vi "Main.vi"() -> ()   [LabVIEW 2020]
panel:
  out "Processed Stream":T1(plugin-control)
  out "Cat 6":dbl(slide) caption="40cm<" scale=0.0..100.0 scale format="%#.3f"
  out "Cat 5":dbl(slide) caption="30-40cm" scale=0.0..100.0 scale format="%#.3f"
  out "Cat 4":dbl(slide) caption="15-30cm" scale=0.0..100.0 scale format="%#.3f"
  out "Cat 3":dbl(slide) caption="10-15cm" scale=0.0..100.0 scale format="%#.3f"
  out "Cat 2":dbl(slide) caption="5-10cm" scale=0.0..100.0 scale format="%#.3f"
  out "Cat 1":dbl(slide) caption="0-5cm" scale=0.0..100.0 scale format="%#.3f"
  out "Live Stream":T1(plugin-control)
  out "Date & Time":string
  in  "Abort":bool
  in  "Maintenance":bool
  in  "Setting":bool
  in  "Report":bool
  in  "Parameters":bool
  in  "Login":bool
  out "Errors":bool
  out "Warnings":bool
  out "Reject Alarm":bool
  out "Sampler Signal":bool
  out "System Unready":bool
  out "System Ready":bool
  # "Smart Grading System"
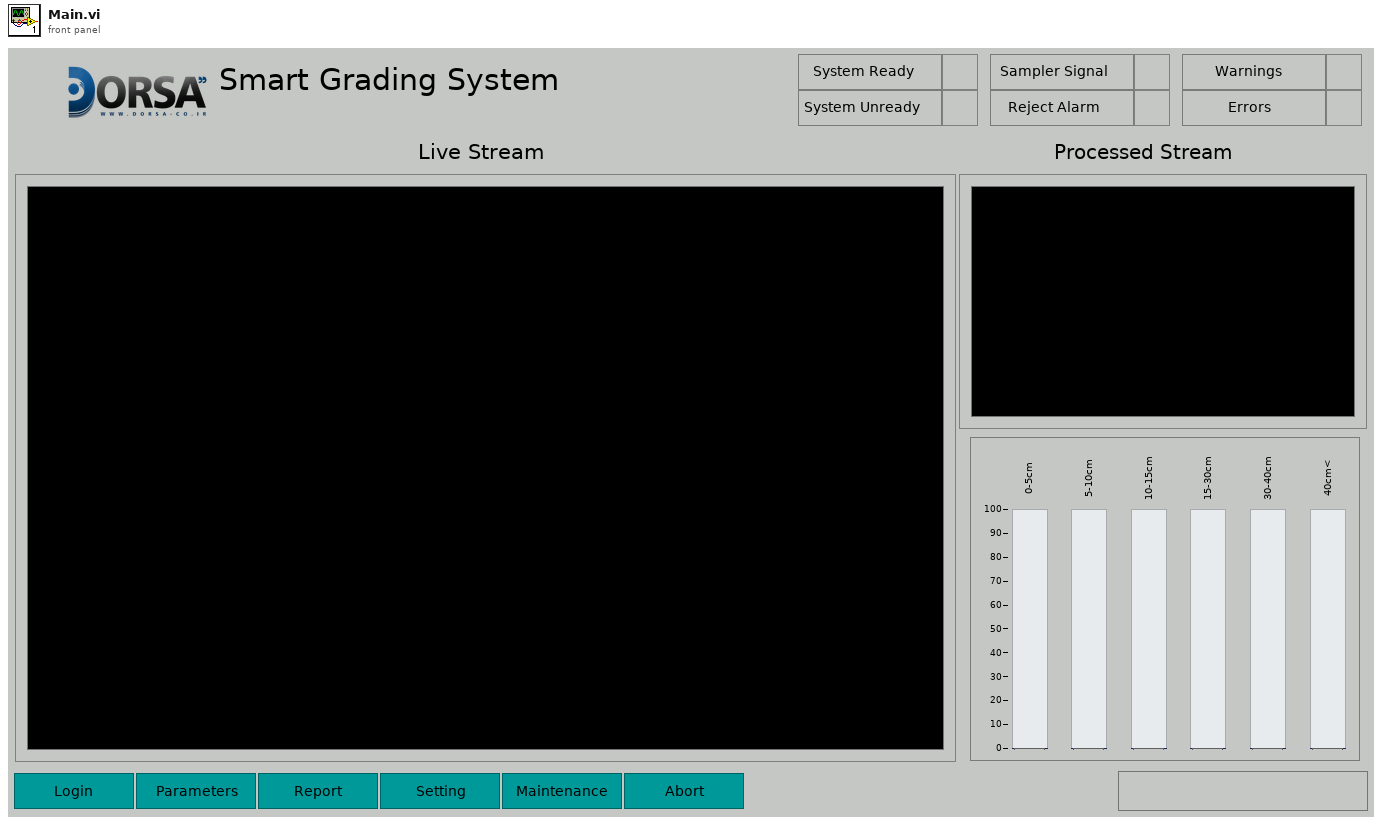
[diagram p1: front panel]
types:
  T1 = typedef "IMAQ Image.ctl" = refnum<image>
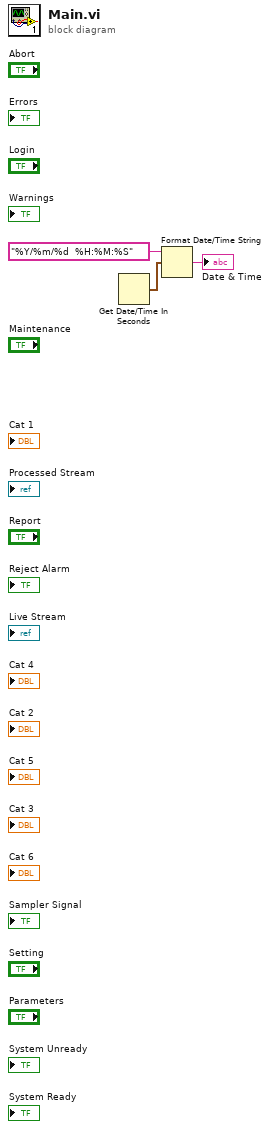
[diagram p0: block diagram]
diagram:
  n1 = Get Date/Time In Seconds() -> (seconds since 1Jan1904=w3:timestamp)
  n2 = Format Date/Time String(time format string (%c)="%Y/%m/%d  %H:%M:%S", seconds (now)=w3) -> (date/time string=→"Date & Time":string)  [unwired: 1 in]
